vi "Calc X & Y Position.vi"(5 "x & y position input array":dbl[](array[numeric]), 6 "Reset X Y":dbl=1.0) -> (2 "phi step":dbl, 14 "y & x traveled output array":dbl[](array[numeric]))   [LabVIEW 2015]
panel:
  out "phi current":dbl
  in  "phi old":dbl
  out "x position":dbl
  out "y position":dbl
  in  "left wheel step (ft)":dbl format="%#_13g"
  in  "right wheel step (ft)":dbl format="%#_13g"
  in  "track width(ft)":dbl=2.5
  in  "X traveled old":dbl format="%#_13g"
  in  "Y traveled old":dbl format="%#_13g"
  in  "distance step":dbl
  out "step y":dbl
  out "step x":dbl
  out "y traveled new":dbl
  out "x traveled new":dbl
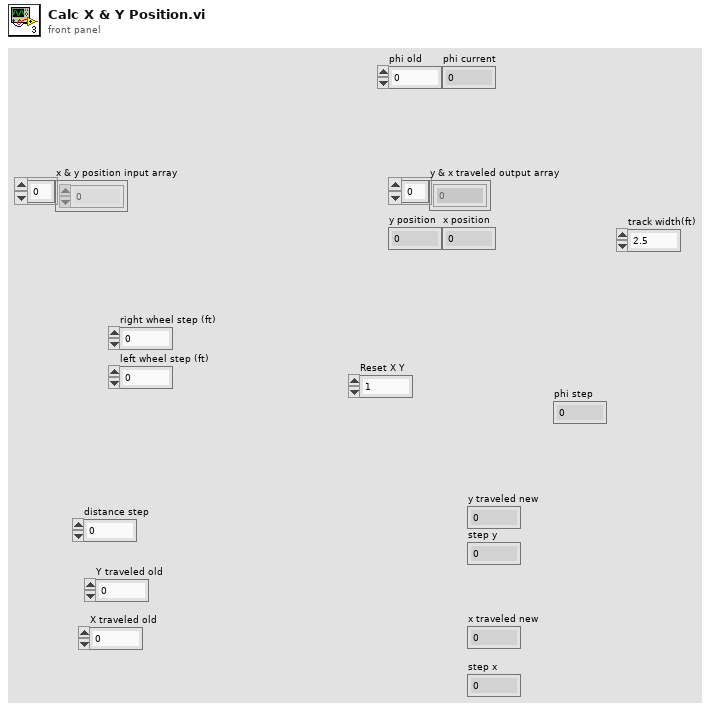
[diagram p1: front panel]
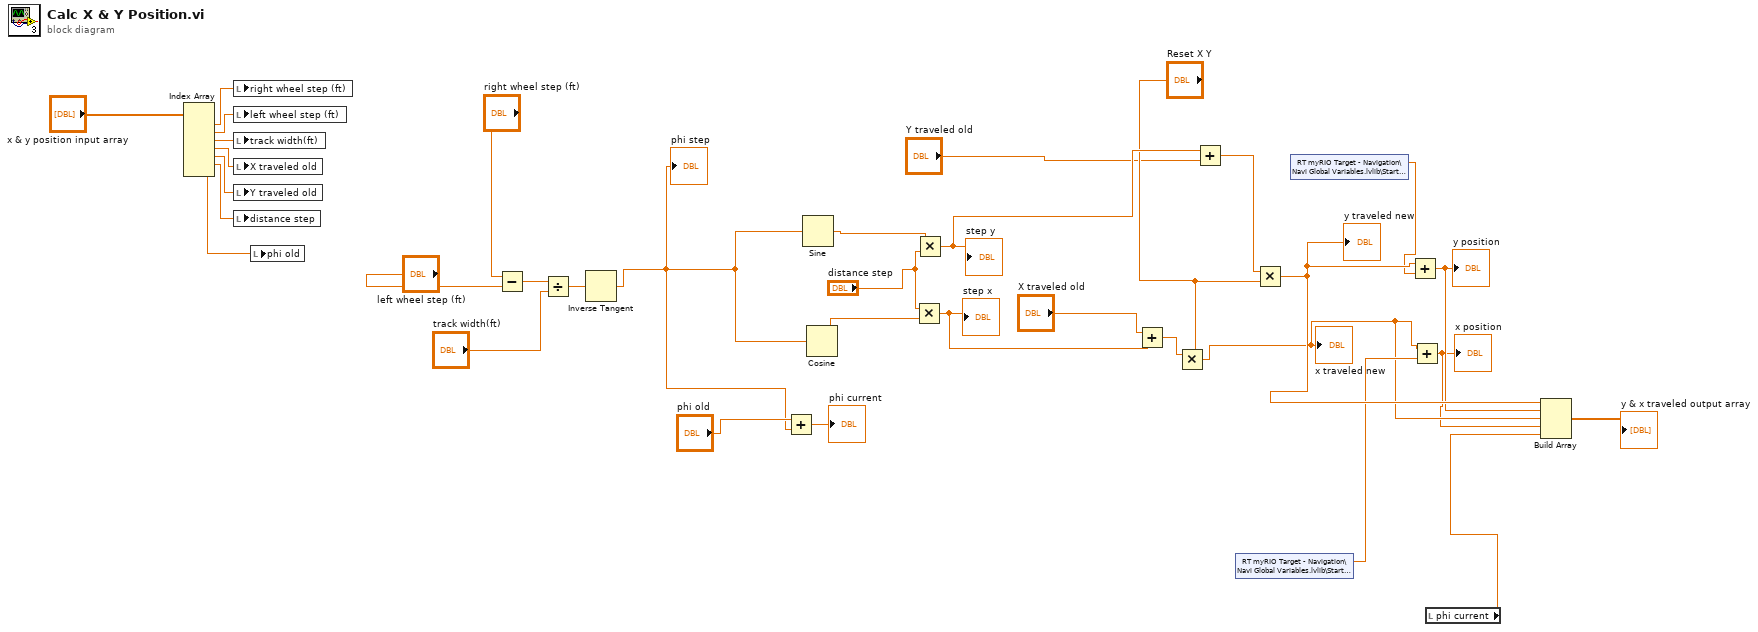
[diagram p0: block diagram]
diagram:
  n1 = Index Array(array="x & y position input array") -> (element #1=w14:dbl, element #2=w11:dbl, element #3=w13:dbl, element #4=w8:dbl, element #5=w7:dbl, element #6=w6:dbl, element #7=w5:dbl)  [unwired: 7 in]
  n2 = local write "right wheel step (ft)"(w14) -> ()
  n3 = local write "left wheel step (ft)"(w11) -> ()
  n4 = local write "track width(ft)"(w13) -> ()
  n5 = local write "X traveled old"(w8) -> ()
  n6 = local write "Y traveled old"(w7) -> ()
  n7 = local write "distance step"(w6) -> ()
  n8 = local write "phi old"(w5) -> ()
  n9 = Subtract(x="right wheel step (ft)", y="left wheel step (ft)") -> (x-y=w30:dbl)
  n10 = Divide(x=w30, y="track width(ft)") -> (x/y=w29:dbl)
  n11 = Inverse Tangent(1:w29) -> (0:w3:dbl)
  "phi step" <- w3
  n12 = Add(x="phi old", y=w3) -> (x+y=→"phi current":dbl)
  n13 = Sine(x=w3) -> (sin(x)=w31:dbl)
  n14 = Cosine(x=w3) -> (cos(x)=w32:dbl)
  n15 = Multiply(x="distance step", y=w32) -> (x*y=w34:dbl)
  "step x" <- w34
  n16 = Multiply(x=w31, y="distance step") -> (x*y=w33:dbl)
  "step y" <- w33
  n17 = Add(x="X traveled old", y=w34) -> (x+y=w27:dbl)
  n18 = Multiply(x=w27, y="Reset X Y") -> (x*y=w19:dbl)
  "x traveled new" <- w19
  n19 = Add(x=w33, y="Y traveled old") -> (x+y=w26:dbl)
  n20 = shared-variable "RT myRIO Target - Navigation\\Navi Global Variables.lvlib\\Start Position X"() -> (w21:dbl)  [unwired: 1 in, 1 out]
  n21 = Multiply(x=w26, y="Reset X Y") -> (x*y=w23:dbl)
  "y traveled new" <- w23
  n22 = shared-variable "RT myRIO Target - Navigation\\Navi Global Variables.lvlib\\Start Position Y"() -> (w22:dbl)  [unwired: 1 in, 1 out]
  n23 = Add(x=w23, y=w22) -> (x+y=w20:dbl)
  "y position" <- w20
  n24 = Add(x=w19, y=w21) -> (x+y=w18:dbl)
  "x position" <- w18
  n25 = local read "phi current"() -> (w1:dbl)
  n26 = Build Array(w23, w20, w19, w18, w1) -> (→"y & x traveled output array":dbl[])
